vi "Test TreeDirectory.vi"() -> ()   [LabVIEW 2026, in "TreeDirectoryExt.lvclass"]
doc: "<b> </b> <b> </b>\n©2016 Q Software Innovations, LLC (QSI)\nwritten by Quentin Alldredge\nproduced in LabVIEW 2015\n\nsupport@qsoftwareinnovations.com\nwww.qsoftwareinnovations.com\n\nAll rights reserved.\n\nRedistribution and use in source and binary forms, with or without modification, are permitted provided that the following conditions are met:\n\n * Redistributions of source code must retain the above copyright notice, this list of conditions and the following disclaimer.\n * Redistributions in binary form must reproduce the above copyright notice, this list of conditions and the following disclaimer in the documentation and/or other materials provided with the distribution.\n * Neither the name of Q Software Innovations, LLC. nor the names of its contributors may be used to endorse or promote products derived from this software without specific prior written permission.\n\nTHIS SOFTWARE IS PROVIDED BY THE COPYRIGHT HOLDERS AND CONTRIBUTORS \"AS IS\" AND ANY EXPRESS OR IMPLIED WARRANTIES, INCLUDING, BUT NOT LIMITED TO, THE IMPLIED WARRANTIES OF MERCHANTABILITY AND FITNESS FOR A PARTICULAR PURPOSE ARE DISCLAIMED. IN NO EVENT SHALL THE COPYRIGHT OWNER OR CONTRIBUTORS BE LIABLE FOR ANY DIRECT, INDIRECT, INCIDENTAL, SPECIAL, EXEMPLARY, OR CONSEQUENTIAL DAMAGES (INCLUDING, BUT NOT LIMITED TO, PROCUREMENT OF SUBSTITUTE GOODS OR SERVICES; LOSS OF USE, DATA, OR PROFITS; OR BUSINESS INTERRUPTION) HOWEVER CAUSED AND ON ANY THEORY OF LIABILITY, WHETHER IN CONTRACT, STRICT LIABILITY, OR TORT (INCLUDING NEGLIGENCE OR OTHERWISE) ARISING IN ANY WAY OUT OF THE USE OF THIS SOFTWARE, EVEN IF ADVISED OF THE POSSIBILITY OF SUCH DAMAGE."
uses:
  TreeDirectoryExt.lvclass
  TreeDirectoryExt.lvclass/TreeDirectoryExt.ctl
  <vilib>/QSI/QControls/QControl Classes/TreeControl/TreeControl.lvclass
panel:
  in  "Tree 2":string(tree)
  in  "Tree":string(tree)
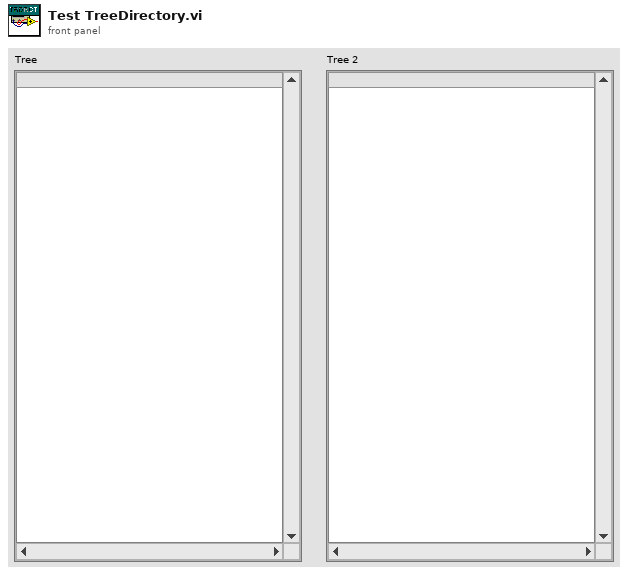
[diagram p1: front panel]
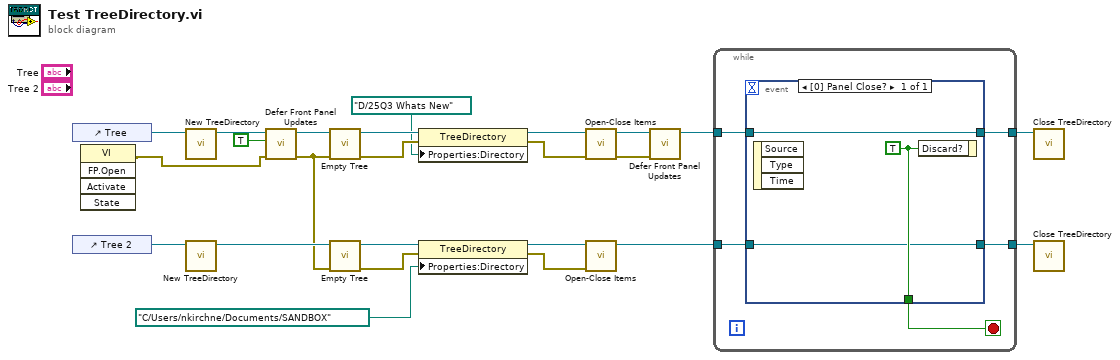
[diagram p0: block diagram]
diagram:
  n1 = control-ref of="Tree"() -> (w15:refnum<vi>)
  n2 = control-ref of="Tree 2"() -> (w12:refnum<vi>)
  n3 = invoke class="VI" method="FP.Open"() -> (error out=w5:errorcluster)  [unwired: 5 in, 4 out]
  n4 = call "New TreeDirectory.vi"("Reference"=w15) -> ("TreeDirectory out"=w14:refnum<class "TreeDirectoryExt.lvclass">)  [unwired: 9 in, 1 out]
  n5 = call "New TreeDirectory.vi"("Reference"=w12) -> ("TreeDirectory out"=w13:refnum<class "TreeDirectoryExt.lvclass">)  [unwired: 9 in, 1 out]
  n6 = call <vilib>:"Defer Front Panel Updates.vi"("error in (no error)"=w5, "Defer Panel Updates (F)"=TRUE, "Tree in"=w14) -> ("error out"=w6:errorcluster, "Tree (dup)"=w23:refnum<class "TreeDirectoryExt.lvclass">)  [unwired: 7 in]
  n7 = call <vilib>:"Empty Tree.vi"("error in (no error)"=w6, "Tree in"=w23) -> ("error out"=w20:errorcluster, "Tree (dup)"=w4:refnum<class "TreeDirectoryExt.lvclass">)  [unwired: 8 in]
  n8 = call <vilib>:"Empty Tree.vi"("error in (no error)"=w6, "Tree in"=w13) -> ("error out"=w10:errorcluster, "Tree (dup)"=w2:refnum<class "TreeDirectoryExt.lvclass">)  [unwired: 8 in]
  n9 = property class="TreeDirectory"(reference=w4, error in=w20, "Properties:Directory"=path "D:/25Q3 Whats New" ("Path")) -> (reference out=w24:refnum<class "TreeDirectoryExt.lvclass">, error out=w19:errorcluster)
  n10 = property class="TreeDirectory"(reference=w2, error in=w10, "Properties:Directory"=path "C:/Users/nkirchne/Documents/SANDBOX" ("Path")) -> (reference out=w8:refnum<class "TreeDirectoryExt.lvclass">, error out=w11:errorcluster)
  n11 = call-dynamic "Open-Close Items.vi"("error in (no error)"=w19, "Tree in"=w24) -> ("error out"=w18:errorcluster, "Tree (dup)"=w21:refnum<class "TreeDirectoryExt.lvclass">)  [unwired: 8 in]
  n12 = call-dynamic "Open-Close Items.vi"("error in (no error)"=w11, "Tree in"=w8) -> ("Tree (dup)"=w9:refnum<class "TreeDirectoryExt.lvclass">)  [unwired: 8 in, 1 out]
  n13 = call <vilib>:"Defer Front Panel Updates.vi"("error in (no error)"=w18, "Tree in"=w21) -> ("Tree (dup)"=w16:refnum<class "TreeDirectoryExt.lvclass">)  [unwired: 8 in, 1 out]
  n14 = while {
    tunnel: [w28] -> w17
    tunnel: w16 -> [w27]
    tunnel: w9 -> [w26]
    tunnel: [w25] -> w7
    stop <- w29 stop-if-true
    n15 = event shown="[0] Panel Close?" {
      selector: _ -> [_]
      dyn-events: _ -> [_]
      timeout: _ -> [_]
      tunnel: [w32] -> w29
      tunnel: [w31] -> w28
      tunnel: w27 -> [w31]
      tunnel: w26 -> [w30]
      tunnel: [w30] -> w25
      event Panel Close? {
        w32 = TRUE ("Discard?")
        n16 = event-data() -> ()  [unwired: 1 in, 3 out]
        n17 = event-data("Discard?"=w32) -> ()  [unwired: 1 in, 1 out]
      }
    }
  }
  n18 = call "Close TreeDirectory.vi"("TreeDirectory in"=w17) -> ()  [unwired: 9 in, 2 out]
  n19 = call "Close TreeDirectory.vi"("TreeDirectory in"=w7) -> ()  [unwired: 9 in, 2 out]
